vi "GetTarget.vi"(8 "error in (no error)":errorcluster, 11 "Instrument.VRM in":refnum<class "Instrument.OxfordVRM.lvclass">) -> (0 "error out":errorcluster, 1 "Target Field Rate (T/min)":dbl[](array[numeric]), 2 "Target Field (T)":dbl[](array[numeric]), 3 "Instrument.VRM out":refnum<class "Instrument.OxfordVRM.lvclass">)   [LabVIEW 2019, in "Instrument.OxfordVRM.lvclass"]
uses:
  Instrument.OxfordVRM.lvclass
  Typedefs/Instrument.VRM.protectedCommands-enum.ctl
  95fe7440-d3b5-4b88-bf75-bf5bcf6ac4e6.vi
  Typedefs/Instrument.VRM.GetTarget--cluster.ctl
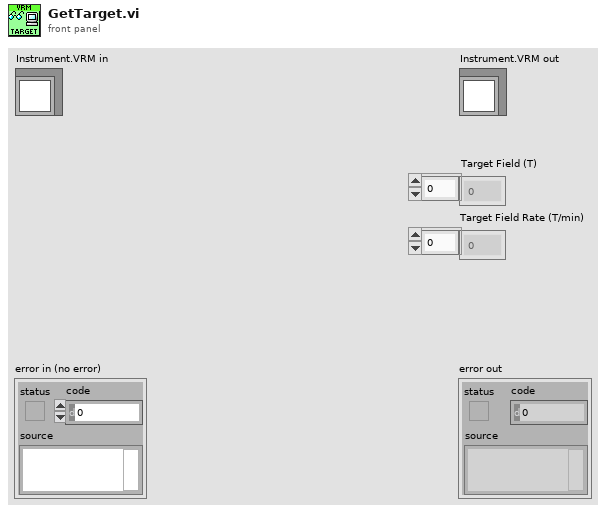
[diagram p1: front panel]
types:
  T1 = typedef "Instrument.OxfordVRM.lvclass/Instrument.VRM.GetTarget--cluster.ctl" = cluster{"field":dbl[], "rate":dbl[]}
  T2 = typedef "Instrument.OxfordVRM.lvclass/Instrument.VRM.protectedCommands-enum.ctl" = enum16{"Hold", "RampToSet", "RampToZero", "Clamp", "SetTarget", "GetStatus", "GetTarget", "GetField"}
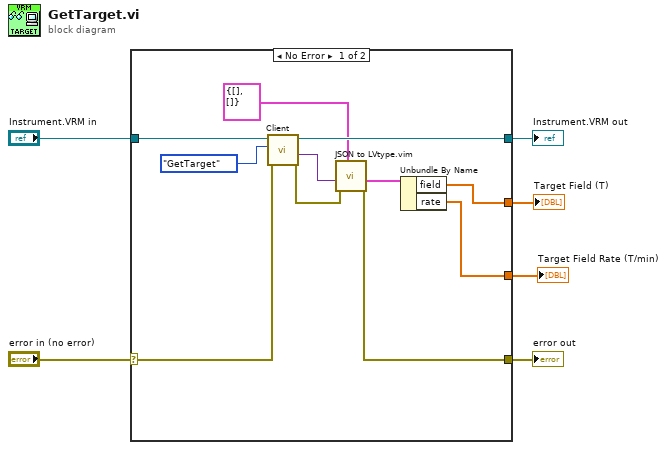
[diagram p0: block diagram]
diagram:
  n1 = case shown="No Error" "error in (no error)" {
    selector: "error in (no error)" -> [w10 w19]
    tunnel: [w11 w19] -> w5
    tunnel: [w14 w18] -> w3
    tunnel: "Instrument.VRM in" -> [w15 w18]
    tunnel: [w8 _] -> w1
    tunnel: [w7 _] -> w2
    frame No Error {
      n2 = call-dynamic "Client.vi"("error in (no error)"=w10, "Command in"=Instrument.VRM.protectedCommands-enum."GetTarget" ("protectedCommands"), "Instrument in"=w15) -> ("error out"=w12:errorcluster, "Data out"=w16:variant, "Instrument out"=w14:refnum<class "Instrument.OxfordVRM.lvclass">)  [unwired: 5 in, 1 out]
      n3 = call "JSON to LVtype.vim"("type"=T1 {"field"=[], "rate"=[]} ("GetTarget"), "error in (no error)"=w12, "JSON Data in"=w16) -> ("error out"=w11:errorcluster, "Data out"=w9:T1)  [unwired: 7 in]
      n4 = Unbundle By Name(w9) -> ("field"=w8:dbl[], "rate"=w7:dbl[])
    }
    frame Error {
    }
  }
  "error out" <- w5
  "Instrument.VRM out" <- w3
  "Target Field (T)" <- w1
  "Target Field Rate (T/min)" <- w2
